vi "Obtain Recipient.vi"(8 "error in (no error)":errorcluster, 11 "Network Endpoint in":refnum<class "Network Endpoint.lvclass">) -> (0 "error out":errorcluster, 2 "Recipient Enqueuer":refnum<class "Message Enqueuer.lvclass">, 3 "Network Endpoint out":refnum<class "Network Endpoint.lvclass">)   [LabVIEW 2020, in "Network Endpoint.lvlib" / "Network Endpoint.lvclass"]
doc: "Override this method to obtain the enqueuer to which your endpoint should forward messages it receives from its remote counterpart."
uses:
  Network Endpoint.lvclass
  <vilib>/ActorFramework/Message Enqueuer/Message Enqueuer.lvclass
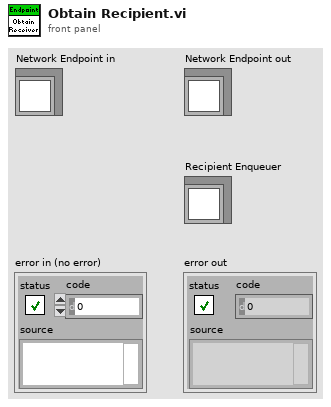
[diagram p1: front panel]
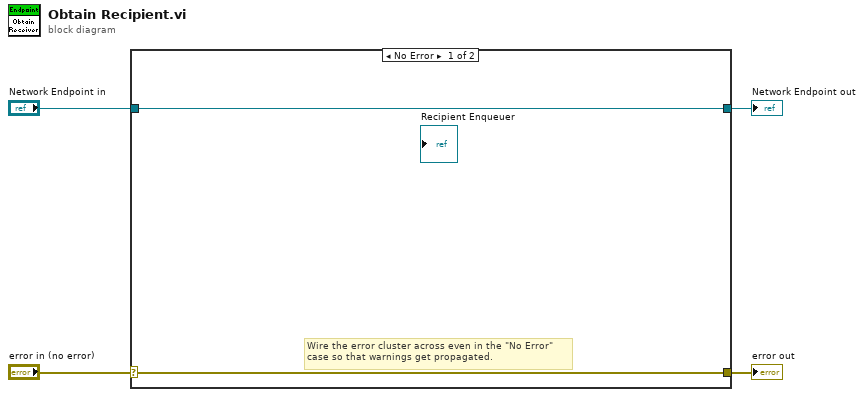
[diagram p0: block diagram]
diagram:
  n1 = case shown="No Error" "error in (no error)" {
    selector: "error in (no error)" -> [w5 w8]
    tunnel: [w5 w8] -> w3
    tunnel: [w6 w7] -> w1
    tunnel: "Network Endpoint in" -> [w6 w7]
    frame No Error {
      # "Wire the error cluster across even in the \"No Error\"\ncase so that warnings get propagated."
    }
    frame Error {
    }
  }
  "error out" <- w3
  "Network Endpoint out" <- w1
